vi "CreatePublicEvents.vi"(8 "error in (no error)":errorcluster, 11 "Microscope":refnum<class "Microscope.lvclass">) -> (0 "error out":errorcluster, 3 "Microscope out":refnum<class "Microscope.lvclass">)   [LabVIEW 2015, in "Microscope.lvclass"]
doc: "---------------------------------------------------------------\nJKI State Machine Objects™\nhttp://jki.net/state-machine-objects/\nCopyright (C) 2005-2015, JKI <info@jki.net>\nALL RIGHTS RESERVEDJKI State Machine Objects (SMO) 1.0.0.5\nJKI - JKI\nCopyright (c) 2016, JKI"
uses:
  Microscope.lvclass
  Typedefs/ValueChanged--EventData--Cluster.ctl
  Microscope.lvclass/Microscope.ctl
  Typedefs/PublicEvents--Microscope.Initialized.ctl
  <vilib>/JKI/JKI SMO/SMO/SMO.lvclass
panel:
  # "For instructions on how to use the JKI State Machine Objects, examples and video tutorials, visit:\nhttp://jki.net/state-machine-objects/\n\nJKI State Machine Objects™\nhttp://jki.net/state-machine-objects/\nCopyright (C) 2005-2015, JKI <info@jki.net>\nALL RIGHTS RESERVED"
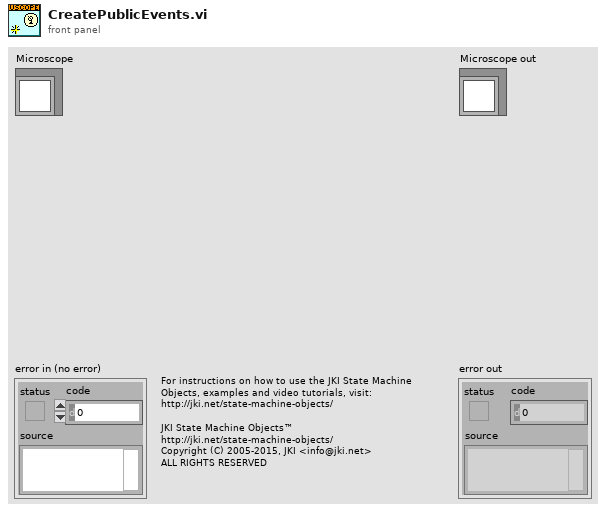
[diagram p1: front panel]
types:
  T1 = typedef "Microscope.lvclass/ValueChanged--EventData--Cluster.ctl" = cluster{"New Value":string}
  T2 = typedef "Microscope.lvclass/PrivateData--Ref.ctl" = refnum<data-value>
  T3 = typedef "Microscope.lvclass/PublicEvents--Microscope.Initialized.ctl" = bool
  T4 = typedef "Microscope.lvclass/PrivateData--Cluster.ctl" = cluster{"Public Events":T5, "Protected Events":T6, "Private Events":T7, "Value":T8, "Dependencies":T9, "Configuration":T10}
  T5 = typedef "Microscope.lvclass/PublicEvents--Cluster.ctl" = cluster{"Value Changed":refnum<user-event>, "Initialized":refnum<user-event>}
  T6 = typedef "Microscope.lvclass/ProtectedEvents--Cluster.ctl" = cluster{"placeholder":refnum<user-event>}
  T7 = typedef "Microscope.lvclass/PrivateEvents--Cluster.ctl" = cluster{"New Value":refnum<user-event>, "Initialize":refnum<user-event>, "CaptureImageAtPosition":refnum<user-event>}
  T8 = typedef "Microscope.lvclass/Value.ctl" = string
  T9 = typedef "Microscope.lvclass/Dependencies--Cluster.ctl" = cluster{"XYStage":refnum<class "XYStage.lvclass">, "Camera":refnum<class "Camera.lvclass">}
  T10 = typedef "Microscope.lvclass/Configuration--Cluster.ctl" = cluster{"XY Stage":string, "Camera":string}
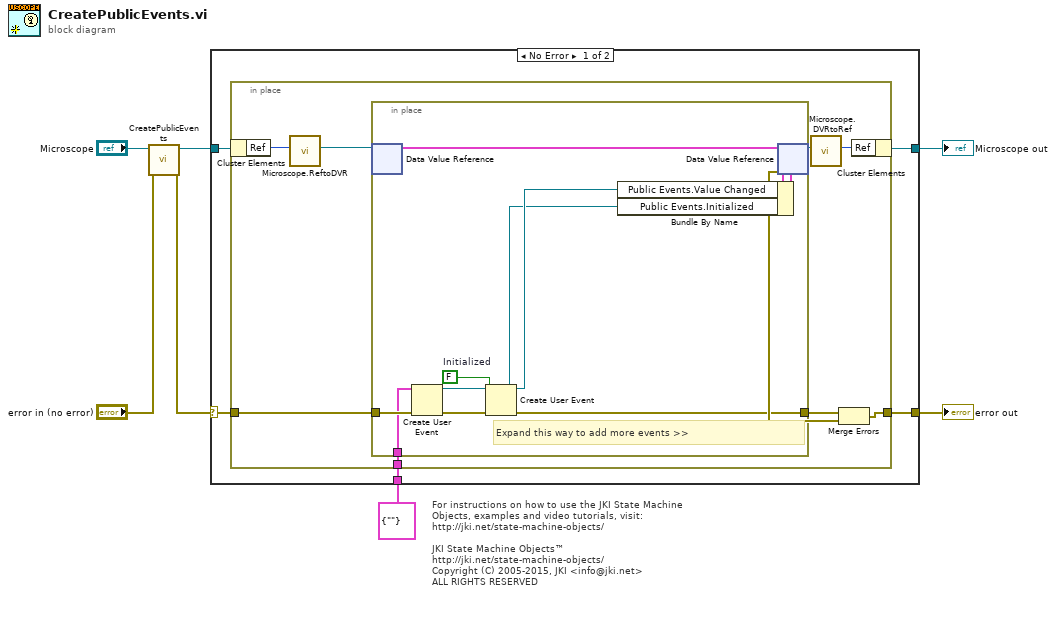
[diagram p0: block diagram]
diagram:
  # "For instructions on how to use the JKI State Machine Objects, examples and video tutorials, visit:\nhttp://jki.net/state-machine-objects/\n\nJKI State Machine Objects™\nhttp://jki.net/state-machine-objects/\nCopyright (C) 2005-2015, JKI <info@jki.net>\nALL RIGHTS RESERVED"
  n1 = call-parent "CreatePublicEvents.vi"("error in (no error)"="error in (no error)", "SMO"="Microscope") -> ("error out"=w1:errorcluster, "SMO out"=w3:refnum<class "Microscope.lvclass">)  [unwired: 8 in]
  n2 = case shown="No Error" w1 {
    selector: w1 -> [w10 w32]
    tunnel: [w9 w32] -> w6
    tunnel: [w11 w31] -> w7
    tunnel: w3 -> [w12 w31]
    tunnel: T1 {"New Value"=""} ("Data In Event Data") -> [w8 _]
    frame No Error {
      n3 = in-place {
        in-place-border: w10 -> [w21]
        in-place-border: [w18] -> w9
        in-place-border: w8 -> [w17]
        n4 = in-place-cluster #1(w12) -> ("Ref"=w16:u32)
        n5 = call "Microscope.ReftoDVR.vi"("Ref"=w16) -> ("Ref"=w15:T2)  [unwired: 10 in]
        n6 = in-place {
          in-place-border: w21 -> [w27]
          in-place-border: [w24] -> w20
          in-place-border: w17 -> [w26]
          w23 = T3 FALSE  # Initialized
          # "Expand this way to add more events >>"
          n7 = in-place-dvr #2(w15) -> (w29:T4)  [unwired: 1 out]
          n8 = Create User Event(user event datatype=w26, error in=w27) -> (user event=w25:refnum<user-event>, error out=w28:errorcluster)
          n9 = Create User Event(user event datatype=w23, error in=w28) -> (user event=w22:refnum<user-event>, error out=w24:errorcluster)
          n10 = Bundle By Name(cluster=w29, "Public Events.Value Changed"=w25, "Public Events.Initialized"=w22) -> (w30:T4)
          n11 = in-place-dvr #2(w30) -> (w14:T2, w19:errorcluster)
        }
        n12 = call "Microscope.DVRtoRef.vi"("Ref"=w14) -> ("Ref"=w13:u32)  [unwired: 10 in]
        n13 = Merge Errors(w20, w19) -> (w18:errorcluster)
        n14 = in-place-cluster #1("Ref"=w13) -> (w11:refnum<class "Microscope.lvclass">)
      }
    }
    frame Error {
    }
  }
  "error out" <- w6
  "Microscope out" <- w7
